vi "Read Voltage.vi"(8 "Error In":errorcluster, 11 "reference in":refnum<class "Scope Base.lvclass">) -> (0 "Error Out":errorcluster, 2 "Voltage":dbl format="%#_g V", 3 "reference out":refnum<class "Scope Base.lvclass">)   [LabVIEW 2023, in "Scope Base.lvlib" / "Scope Base.lvclass"]
uses:
  Scope Base.lvclass
  D:/git/HAL/HAL GOOP4/Instrument Base/Instrument Base.lvclass
  Interfaces/IConfigure/IConfigure.lvclass
  Instrument Base/Instrument Base.lvclass
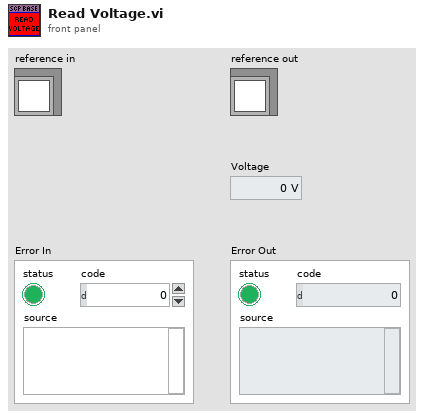
[diagram p1: front panel]
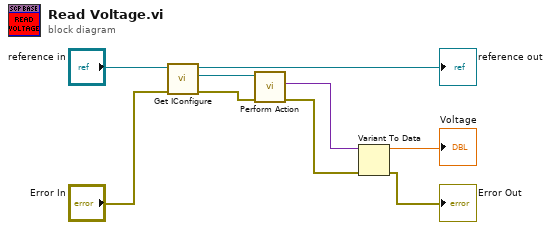
[diagram p0: block diagram]
diagram:
  n1 = call "Get IConfigure.vi"("Error In"="Error In", "reference in"="reference in") -> ("Error Out"=w6:errorcluster, "IConfigure"=w7:refnum<class "IConfigure.lvclass">, "reference out"=→"reference out":refnum<class "Scope Base.lvclass">)  [unwired: 7 in]
  n2 = call-dynamic "Perform Action.vi"("Error In"=w6, "object in"=w7) -> ("Error Out"=w4:errorcluster, "Output"=w5:variant)  [unwired: 7 in, 1 out]
  n3 = Variant To Data(error in=w4, Variant=w5) -> (data=→"Voltage":dbl, error out=→"Error Out":errorcluster)  [unwired: 1 in]
